vi "Theme Colors.vi"() -> ()   [LabVIEW 2018, in "Theme.lvlib"]
uses:
  Theme.lvlib
panel:
  out "Page Text Caption":u32(colorbox)=16777215
  out "Tab Hover X":u32(colorbox)=6710886
  out "Tab Text Inactive":u32(colorbox)=13421772
  out "Tab Text Active":u32(colorbox)=16777215
  out "Tab Hover":u32(colorbox)=6118749
  out "Tab Inactive":u32(colorbox)=4802889
  out "Tab Active":u32(colorbox)=1118481
  out "Tab BG":u32(colorbox)=3355443
  out "Page Mask":u32(colorbox)=3355443
  out "BG":u32(colorbox)=3355443
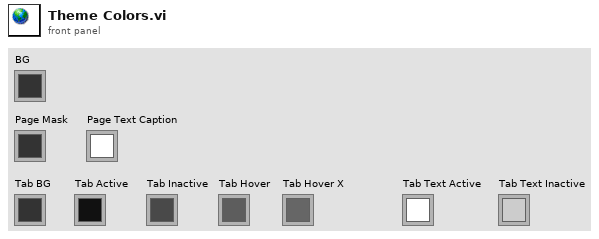
[diagram p1: front panel]
diagram:
